vi "nanoVoltRead.vi"() -> ()   [LabVIEW 2013]
uses:
  <vilib>/Utility/file.llb/Write To Spreadsheet File (string).vi
panel:
  in  "Rate (0.01 - 5)":string
  out "Time (s)":dbl caption="Elapsed Time (s)"
  out "XY Graph":cluster{dbl[], dbl[]}(graph)
  in  "file (use dialog)":path
  out "Measurement Number":i32
  in  "stop":bool
  out "Voltage(V)":dbl
  in  "GPIB\nAddress":string="9"
  # "Keithley Model 2182A Nanovoltmeter Read\n5/21/2012\nMichael Kabatek\nCSU Magnetics Lab"
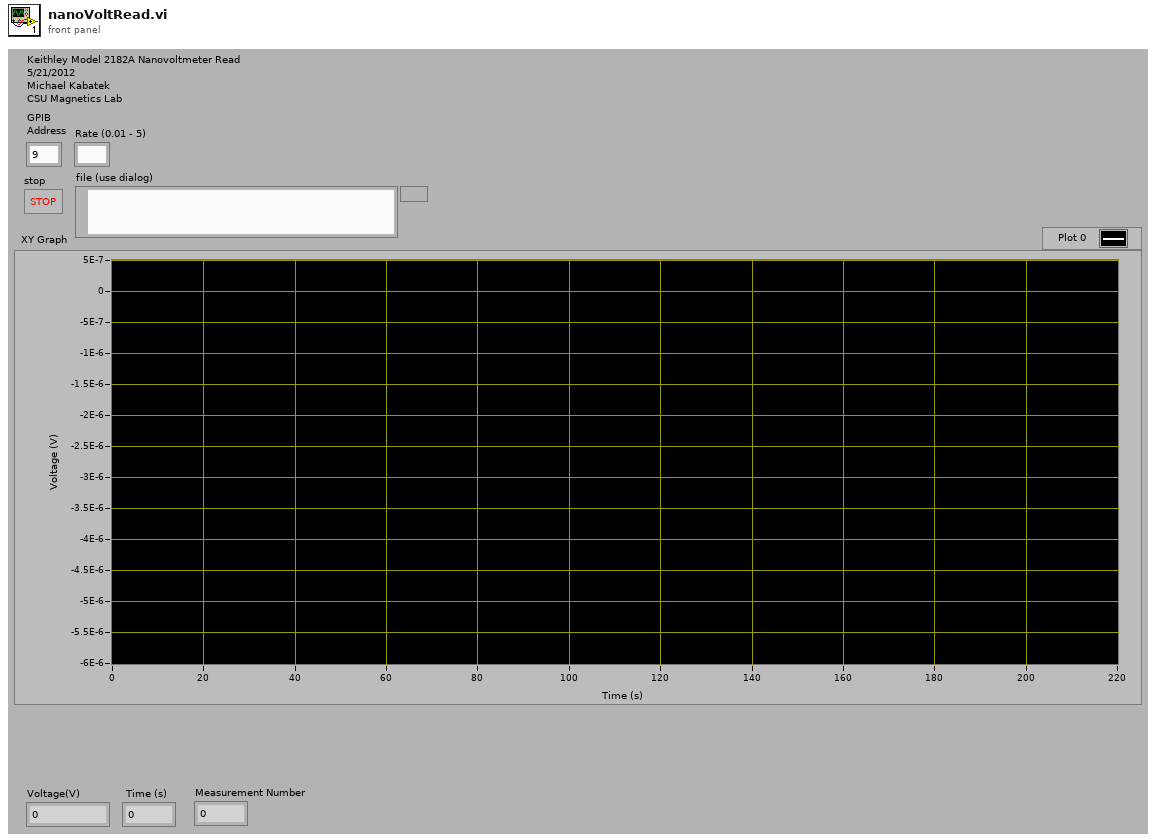
[diagram p1: front panel]
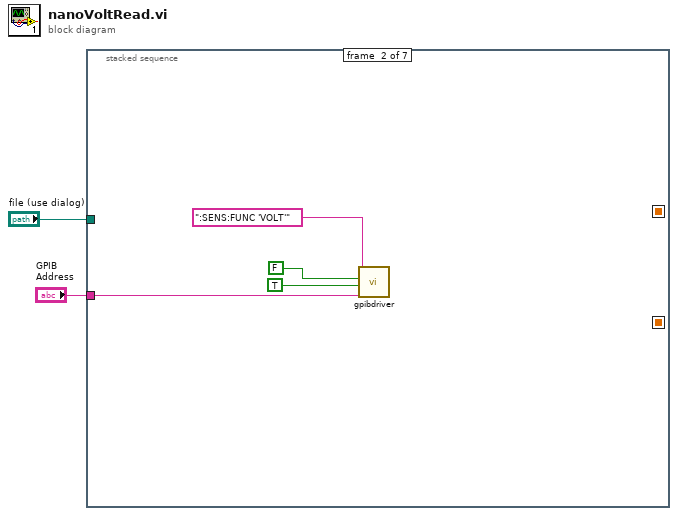
[diagram p0: block diagram]
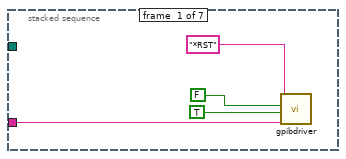
[diagram p2: hidden frame]
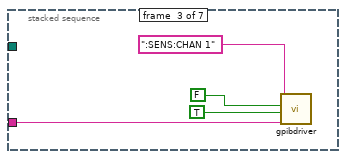
[diagram p3: hidden frame]
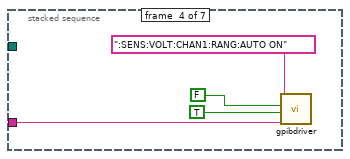
[diagram p4: hidden frame]
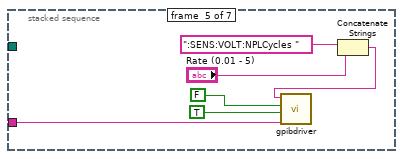
[diagram p5: hidden frame]
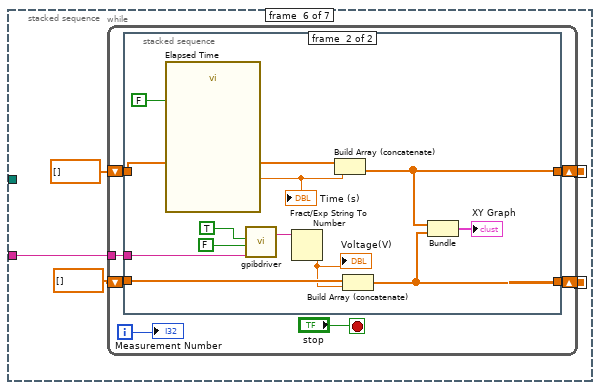
[diagram p6: hidden frame]
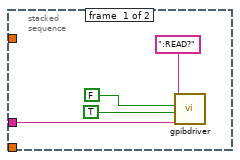
[diagram p7: hidden frame]
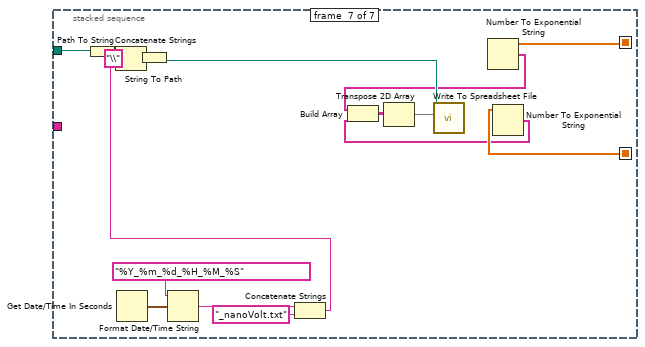
[diagram p8: hidden frame]
diagram:
  n1 = stacked-sequence {
    seq-local: [_ _ _ _ _ w27 _] -> [_ _ _ _ _ _ w59]
    seq-local: [_ _ _ _ _ w25 _] -> [_ _ _ _ _ _ w58]
    tunnel: "GPIB\nAddress" -> [w3 w7 w11 w15 w22 w29 _]
    tunnel: "file (use dialog)" -> [_ _ _ _ _ _ w61]
    frame #0 {
      n2 = call "gpibdriver.vi"("Characters to Write"="*RST", "Read"=FALSE, "Write"=TRUE ("Write 3"), "GPIB\nAddress"=w3) -> ()  [unwired: 2 in, 1 out]
    }
    frame #1 {
      n3 = call "gpibdriver.vi"("Characters to Write"=":SENS:FUNC 'VOLT'", "Read"=FALSE, "Write"=TRUE ("Write 3"), "GPIB\nAddress"=w7) -> ()  [unwired: 2 in, 1 out]
    }
    frame #2 {
      n4 = call "gpibdriver.vi"("Characters to Write"=":SENS:CHAN 1", "Read"=FALSE, "Write"=TRUE ("Write 3"), "GPIB\nAddress"=w11) -> ()  [unwired: 2 in, 1 out]
    }
    frame #3 {
      n5 = call "gpibdriver.vi"("Characters to Write"=":SENS:VOLT:CHAN1:RANG:AUTO ON", "Read"=FALSE, "Write"=TRUE ("Write 3"), "GPIB\nAddress"=w15) -> ()  [unwired: 2 in, 1 out]
    }
    frame #4 {
      n6 = Concatenate Strings(":SENS:VOLT:NPLCycles " ("Characters to Write"), "Rate (0.01 - 5)") -> (w19:string)
      n7 = call "gpibdriver.vi"("Characters to Write"=w19, "Read"=FALSE, "Write"=TRUE ("Write 3"), "GPIB\nAddress"=w22) -> ()  [unwired: 2 in, 1 out]
    }
    frame #5 {
      n8 = while {
        tunnel: w29 -> [w36]
        shift-right: [w34] -> w27
        shift-left: dbl[] [] -> [w33]
        shift-right: [w30] -> w25
        shift-left: dbl[] [] -> [w31]
        i -> [w32]
        stop <- "stop" stop-if-true
        n9 = stacked-sequence {
          tunnel: w36 -> [w37 w50]
          tunnel: [_ w42] -> w34
          tunnel: w33 -> [_ w49]
          tunnel: w31 -> [_ w46]
          tunnel: [_ w43] -> w30
          frame #0 {
            n10 = call "gpibdriver.vi"("Characters to Write"=":READ?", "Read"=FALSE, "Write"=TRUE ("Write 3"), "GPIB\nAddress"=w37) -> ()  [unwired: 2 in, 1 out]
          }
          frame #1 {
            n11 = call "Elapsed Time"("Auto Reset"=FALSE) -> ("Elapsed Time (s)"=w45:dbl)  [unwired: 11 in, 7 out]
            "Time (s)" <- w45
            n12 = call "gpibdriver.vi"("Read"=TRUE, "Write"=FALSE ("Write 3"), "GPIB\nAddress"=w50) -> ("Characters Read"=w47:string)  [unwired: 3 in]
            n13 = Fract/Exp String To Number(string=w47) -> (number=w48:dbl)  [unwired: 3 in, 1 out]
            "Voltage(V)" <- w48
            n14 = Build Array (concatenate)(w46, w45) -> (w43:dbl[])
            n15 = Build Array (concatenate)(w49, w48) -> (w42:dbl[])
            n16 = Bundle(w43, w42) -> (→"XY Graph":cluster{dbl[], dbl[]})  [unwired: 1 in]
          }
        }
        "Measurement Number" <- w32
      }
    }
    frame #6 {
      n17 = Path To String(path=w61) -> (string=w64:string)
      n18 = Get Date/Time In Seconds() -> (seconds since 1Jan1904=w68:timestamp)
      n19 = Format Date/Time String(time format string (%c)="%Y_%m_%d_%H_%M_%S", seconds (now)=w68) -> (date/time string=w66:string)  [unwired: 1 in]
      n20 = Concatenate Strings(w66, "_nanoVolt.txt" ("string")) -> (w60:string)
      n21 = Concatenate Strings(w64, "\\" ("string"), w60) -> (w62:string)
      n22 = String To Path(string=w62) -> (path=w57:path)
      n23 = Number To Exponential String(number=w58) -> (E-format string=w53:string[])  [unwired: 3 in]
      n24 = Number To Exponential String(number=w59) -> (E-format string=w54:string[])  [unwired: 3 in]
      n25 = Build Array(w53, w54) -> (w56:string[][])
      n26 = Transpose 2D Array(2D array=w56) -> (transposed array=w55:string[][])
      n27 = call-poly <vilib>:"Write To Spreadsheet File.vi"("2D data"=w55, "file path (dialog if empty)"=w57) -> ()  [unwired: 6 in, 1 out]
    }
  }
